vi "AssertComplex_1DArray-CSG.vi"(8 "error in":errorcluster, 11 "Array":csg[](array[numeric])) -> (0 "error out":errorcluster, 3 "Array":csg[](array[numeric]))   [LabVIEW 2020, in "OpenLvVision_OpenCv.lvlib"]
uses:
  OpenLvVision_OpenCv.lvlib
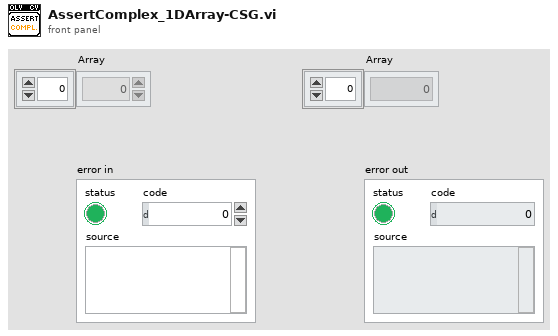
[diagram p1: front panel]
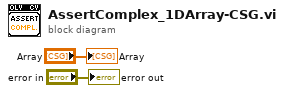
[diagram p0: block diagram]
diagram:
  "error out" <- "error in"
  "Array" <- "Array"
